vi "getValue.vi"(8 "error in (no error)":errorcluster, 11 "tBSONTimestamp in":refnum<class "tBSONTimestamp.lvclass">) -> (0 "error out":errorcluster, 2 "Value":timestamp, 3 "tBSONTimestamp out":refnum<class "tBSONTimestamp.lvclass">)   [LabVIEW 2013, in "BSON.lvlib" / "tBSONTimestamp.lvclass"]
uses:
  tBSONTimestamp.lvclass
  tBSONTimestamp.lvclass/tBSONTimestamp.ctl
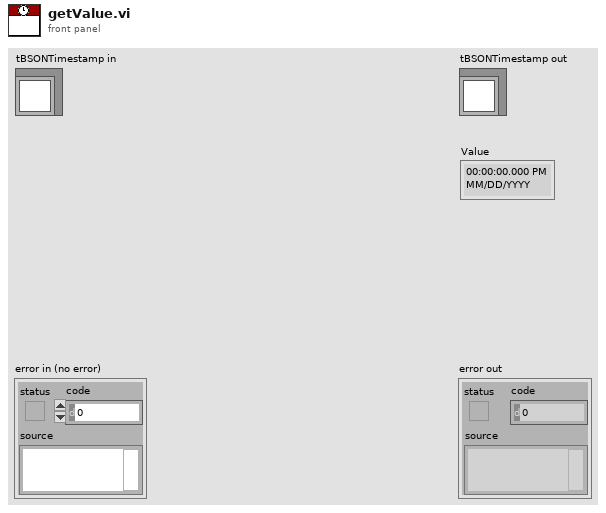
[diagram p1: front panel]
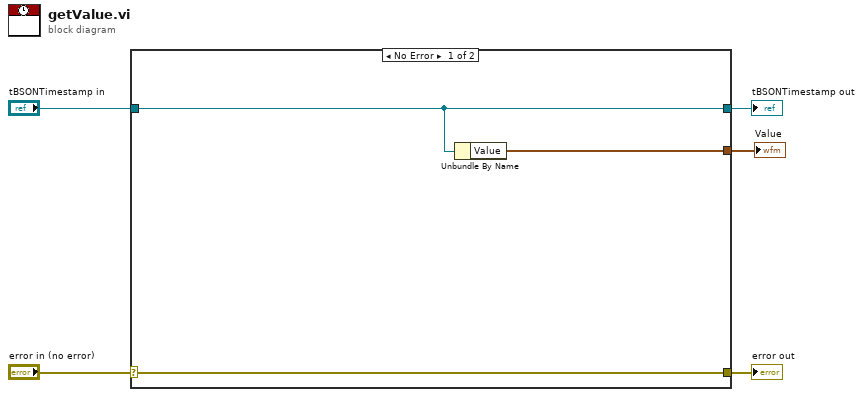
[diagram p0: block diagram]
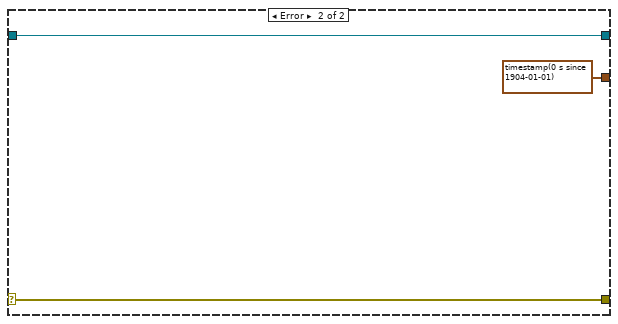
[diagram p2: hidden frame]
diagram:
  n1 = case shown="No Error" "error in (no error)" {
    selector: "error in (no error)" -> [w8 w11]
    tunnel: [w8 w11] -> w4
    tunnel: [w7 w10] -> w2
    tunnel: "tBSONTimestamp in" -> [w7 w10]
    tunnel: [w6 timestamp(0 s since 1904-01-01) ("Value")] -> w1
    frame No Error {
      n2 = Unbundle By Name(w7) -> ("Value"=w6:timestamp)
    }
    frame Error {
    }
  }
  "error out" <- w4
  "tBSONTimestamp out" <- w2
  "Value" <- w1
